vi "LS330_CMD.vi"(8 "error in":errorcluster, 10 "CMD":string, 11 "VISA resource name":refnum<visa-resource-name>) -> (0 "error out":errorcluster, 3 "VISA resource name out":refnum<visa-resource-name>)   [LabVIEW 2021]
uses:
  31ca410e-eb9f-45fd-896e-dea07802b8d0.vi
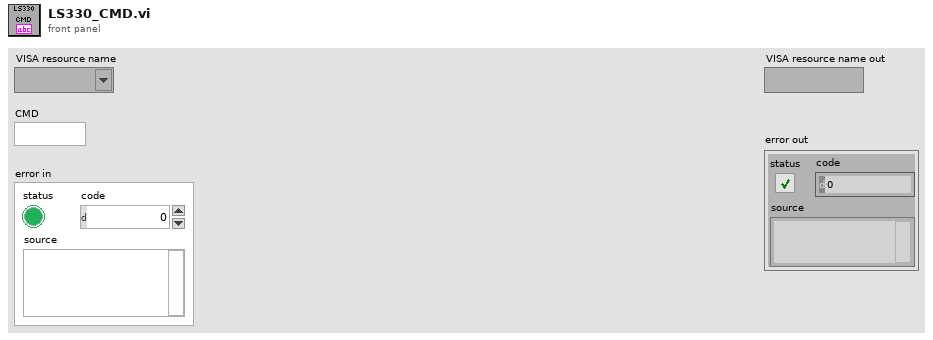
[diagram p1: front panel]
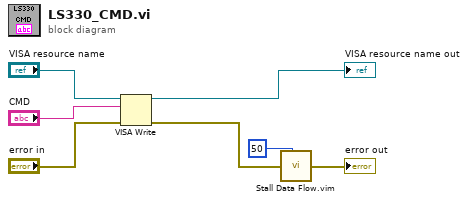
[diagram p0: block diagram]
diagram:
  n1 = VISA Write(VISA resource name="VISA resource name", write buffer="CMD", error in (no error)="error in") -> (VISA resource name out=→"VISA resource name out":refnum<visa-resource-name>, error out=w1:errorcluster)  [unwired: 1 out]
  n2 = call "Stall Data Flow.vim"("value in"=w1, "milliseconds to wait"=u32 50) -> ("value out"=→"error out":errorcluster)  [unwired: 1 out]
